vi "CurrentServoStatus.vi"(2 "New Servo Status":cluster{"mode":string, "position":dbl} {"position" min=0.0 max=180.0 step=1.0}, 3 "Operation":T1) -> (1 "Current Servo Status":cluster{"mode":string, "position":dbl} {"position" min=0.0 max=180.0 step=1.0})   [LabVIEW 2024]
uses:
  DataTypes/OperationTypeForFunctionalGlobalVariable.ctl
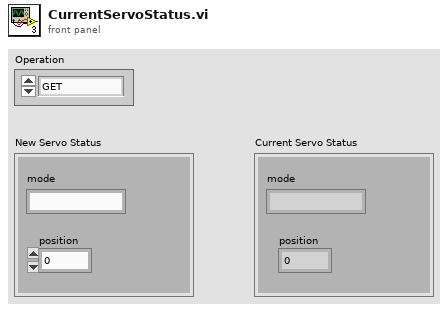
[diagram p1: front panel]
types:
  T1 = typedef "OperationTypeForFunctionalGlobalVariable.ctl" = enum16{"GET", "SET"}
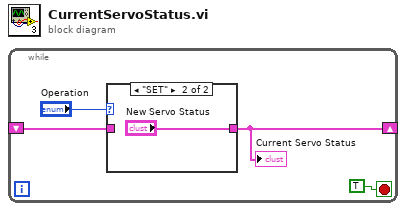
[diagram p0: block diagram]
diagram:
  n1 = while {
    shift-right: [w1] -> _
    shift-left: _ -> [w2]
    stop <- TRUE stop-if-true
    n2 = case shown="\"SET\"" "Operation" {
      tunnel: w2 -> [w5 _]
      tunnel: [w5 "New Servo Status"] -> w1
      frame "GET", Default {
      }
      frame "SET" {
      }
    }
    "Current Servo Status" <- w1
  }
